vi "Format Image Information.vi"(7 "Image Acquisition Parameters Array":T1[](array[typedef]) {"Z Steps Size (um)" min=0.0; "Number of Z Steps" min=1; "Frames Accumulations" min=1; "Frames Per Capture" min=1; "Line Accumulations" min=1; "Image Format" items=["64 x 64"=64, "128 x 128"=128, "256 x 256"=256, "512 x 512"=512, "1024 x 1024"=1024, "2048 x 2048"=2048]}) -> (8 "Result":string)   [LabVIEW 2016]
uses:
  Type Defs/Image Acquisition Parameters.ctl
  Type Defs/JSON Parameters.ctl
panel:
  # "Copyright (C) 2020 Edward S Allgeyer\n\nRedistribution and use in source and binary forms, with or without\nmodification, are permitted provided that the following conditions\nare met:\n\n1. Redistributions of source code must retain the above copyright\n   notice, this list of conditions and the following disclaimer.\n\n2. Redistributions in binary form must reproduce the above copyright\n   notice, this list of conditions and the following disclaimer in\n   the documentation and/or other materials provided with the\n   distribution.\n\n3. Neither the name of the copyright holder nor the names of its\n   contributors may be used to endorse or promote products derived\n   from this software without specific prior written permission.\n\nTHIS SOFTWARE IS PROVIDED BY THE COPYRIGHT HOLDERS AND CONTRIBUTORS\n\"AS IS\" AND ANY EXPRESS OR IMPLIED WARRANTIES, INCLUDING, BUT NOT\nLIMITED TO, THE IMPLIED WARRANTIES OF MERCHANTABILITY AND FITNESS\nFOR A PARTICULAR PURPOSE ARE DISCLAIMED. IN NO EVENT SHALL THE\nCOPYRIGHT HOLDER OR CONTRIBUTORS BE LIABLE FOR ANY DIRECT, INDIRECT,\nINCIDENTAL, SPECIAL, EXEMPLARY, OR CONSEQUENTIAL DAMAGES (INCLUDING,\nBUT NOT LIMITED TO, PROCUREMENT OF SUBSTITUTE GOODS OR SERVICES;\nLOSS OF USE, DATA, OR PROFITS; OR BUSINESS INTERRUPTION) HOWEVER\nCAUSED AND ON ANY THEORY OF LIABILITY, WHETHER IN CONTRACT, STRICT\nLIABILITY, OR TORT (INCLUDING NEGLIGENCE OR OTHERWISE) ARISING IN\nANY WAY OUT OF THE USE OF THIS SOFTWARE, EVEN IF ADVISED OF THE\nPOSSIBILITY OF SUCH DAMAGE."
  # "XY"
  # "Z"
  # "Length"
  # "Height"
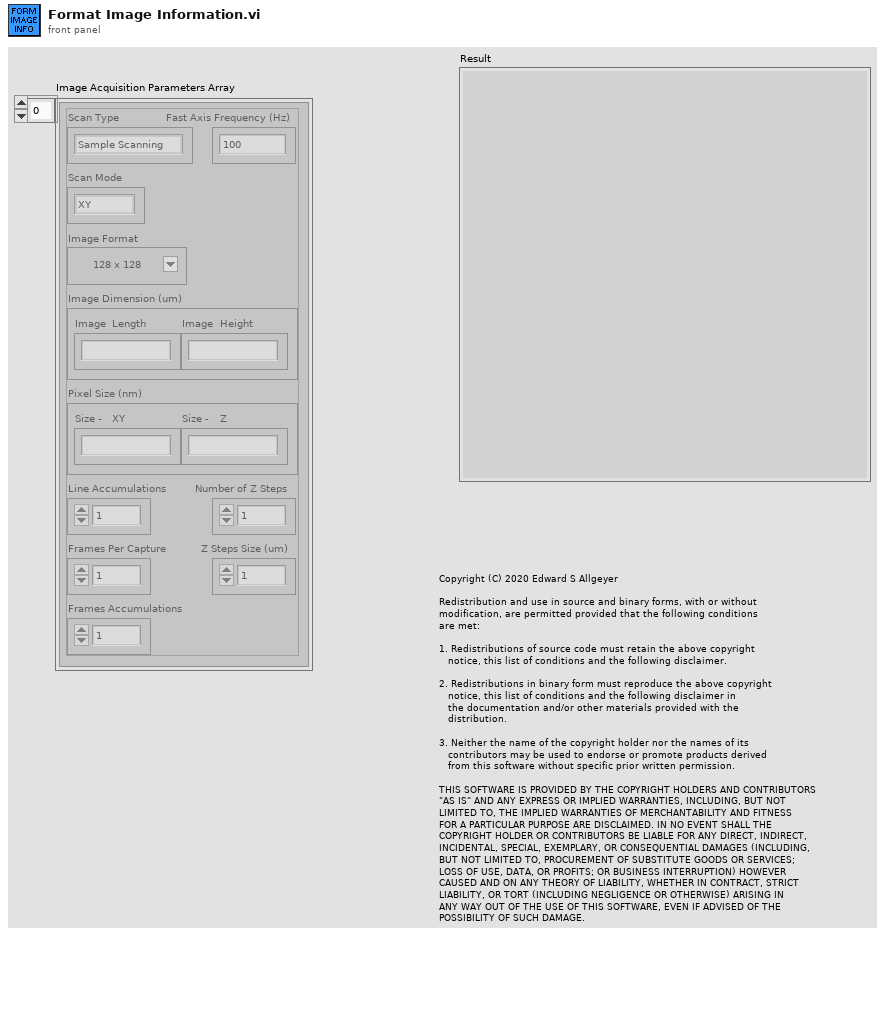
[diagram p1: front panel]
types:
  T1 = typedef "Image Acquisition Parameters.ctl" = cluster{"Scan Type":enum16{"Sample Scanning", "Beam Scanning"}, "Scan Mode":enum16{"XY", "XZ", "YZ", "XYZ"}, "Fast Axis Frequency (Hz)":dbl, "Image Format":u16, "Line Accumulations":u16, "Frames Per Capture":u16, "Frames Accumulations":u16, "Image Dimension (um)":dbl[], "Number of Z Steps":u8, "Z Steps Size (um)":dbl, "Pixel Size (nm)":dbl[]}
  T2 = typedef "JSON Parameters.ctl" = cluster{"Scan Mode":string, "pxHeight":u16, "pxWidth":u16, "umHeight":dbl, "umWidth":dbl, "lineAccums":u16, "framesPerCapture":u16, "numZsteps":u8, "zStepSize_um":dbl, "laser_STED":bool, "laser_656":bool, "laser_485":bool, "laser_405":bool, "laser_whiteLight":bool, "power_STED":dbl, "power_405":dbl, "detector_farRed":bool, "detector_Orange":bool, "detector_Green":bool, "detector_sumAll":bool}
  T3 = typedef "Laser Controls.ctl" = cluster{"STED Power (0-5V)":dbl, "STED":bool, "640 nm":bool, "485 nm":bool, "Manual Control":bool, "White Light":bool, "405 nm":bool, "405 Power (0-5V)":dbl}
  T4 = typedef "Detectors.ctl" = cluster{"PMT":bool, "Far Red (697/75 nm)":bool, "Orange (624/40 nm)":bool, "Green (525/50 nm)":bool, "Sum All":bool}
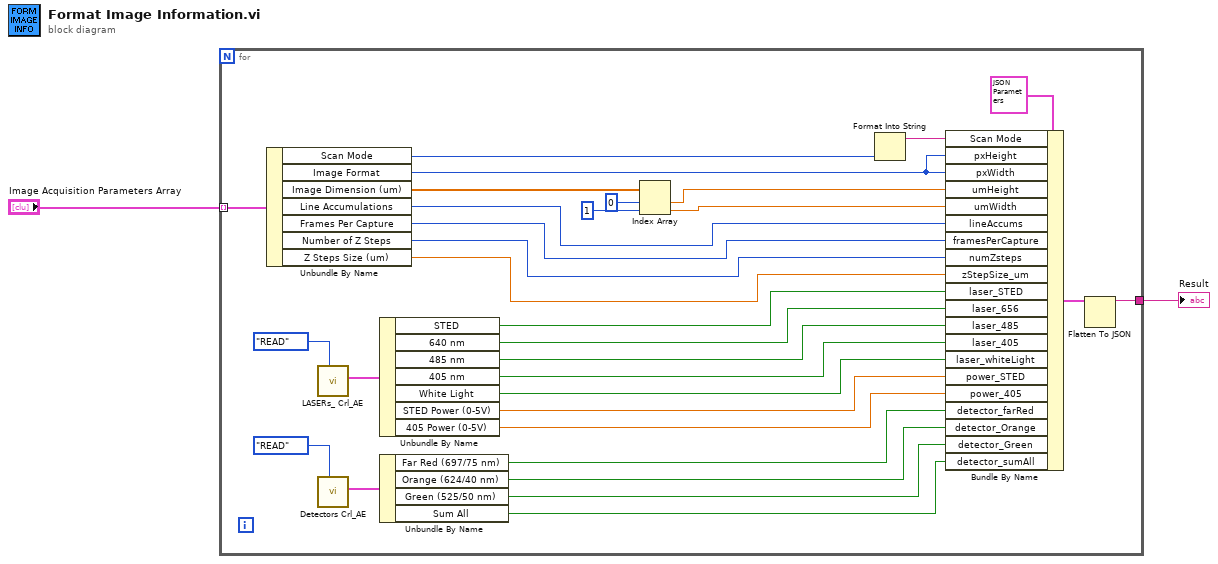
[diagram p0: block diagram]
diagram:
  n1 = for {
    tunnel: "Image Acquisition Parameters Array" -> [w27] mode=indexing
    tunnel: [w14] -> w1
    n2 = Unbundle By Name(w27) -> ("Scan Mode"=w33:enum16{"XY", "XZ", "YZ", "XYZ"}, "Image Format"=w22:u16, "Image Dimension (um)"=w32:dbl[], "Line Accumulations"=w18:u16, "Frames Per Capture"=w17:u16, "Number of Z Steps"=w16:u8, "Z Steps Size (um)"=w15:dbl)
    n3 = call "LASERs_ Crl_AE.vi"("Action"=enum16{"READ", "WRITE"}."READ") -> ("Laser Parameters Out"=w31:T3)  [unwired: 10 in]
    n4 = call "Detectors Crl_AE.vi"("Action"=enum16{"READ", "WRITE"}."READ") -> ("Detectors Parameters Out"=w28:T4)  [unwired: 10 in]
    n5 = Unbundle By Name(w31) -> ("STED"=w13:bool, "640 nm"=w12:bool, "485 nm"=w11:bool, "405 nm"=w10:bool, "White Light"=w9:bool, "STED Power (0-5V)"=w8:dbl, "405 Power (0-5V)"=w7:dbl)
    n6 = Unbundle By Name(w28) -> ("Far Red (697/75 nm)"=w6:bool, "Orange (624/40 nm)"=w5:bool, "Green (525/50 nm)"=w4:bool, "Sum All"=w3:bool)
    n7 = Index Array(array=w32, index #1=0 ("index"), index #2=1 ("index")) -> (element #1=w21:dbl, element #2=w19:dbl)
    n8 = Format Into String(w33) -> (resulting string=w23:string)  [unwired: 3 in, 1 out]
    n9 = Bundle By Name(cluster=T2 {"Scan Mode"="", "pxHeight"=0, "pxWidth"=0, "umHeight"=0.0, "umWidth"=0.0, "lineAccums"=0, "framesPerCapture"=0, "numZsteps"=0, "zStepSize_um"=0.0, "laser_STED"=FALSE, "laser_656"=FALSE, "laser_485"=FALSE, "laser_405"=FALSE, "laser_whiteLight"=FALSE, "power_STED"=0.0, "power_405"=0.0, "detector_farRed"=FALSE, "detector_Orange"=FALSE, "detector_Green"=FALSE, "detector_sumAll"=FALSE} ("img_params"), "Scan Mode"=w23, "pxHeight"=w22, "pxWidth"=w22, "umHeight"=w21, "umWidth"=w19, "lineAccums"=w18, "framesPerCapture"=w17, "numZsteps"=w16, "zStepSize_um"=w15, "laser_STED"=w13, "laser_656"=w12, "laser_485"=w11, "laser_405"=w10, "laser_whiteLight"=w9, "power_STED"=w8, "power_405"=w7, "detector_farRed"=w6, "detector_Orange"=w5, "detector_Green"=w4, "detector_sumAll"=w3) -> (w24:T2)
    n10 = Flatten To JSON(anything=w24) -> (JSON string=w14:string)  [unwired: 2 in, 1 out]
  }
  "Result" <- w1
